vi "Display Results.vi"(8 "error in (no error)":errorcluster, 10 "Results.lvclass":refnum<class "Results.lvclass">, 11 "Operator UI in":refnum<class "Measurement UI.lvclass">) -> (0 "error out":errorcluster, 3 "Operator UI out":refnum<class "Measurement UI.lvclass">)   [LabVIEW 2015, in "Measurement UI.lvlib" / "Measurement UI.lvclass"]
uses:
  Measurement UI.lvclass
  Results/Results.lvclass
  Measurement UI.lvclass/Measurement UI.ctl
  Results/Results.lvclass/Results.ctl
  Accessors/Read Results Listbox.vi
  User Interface/UI.lvclass
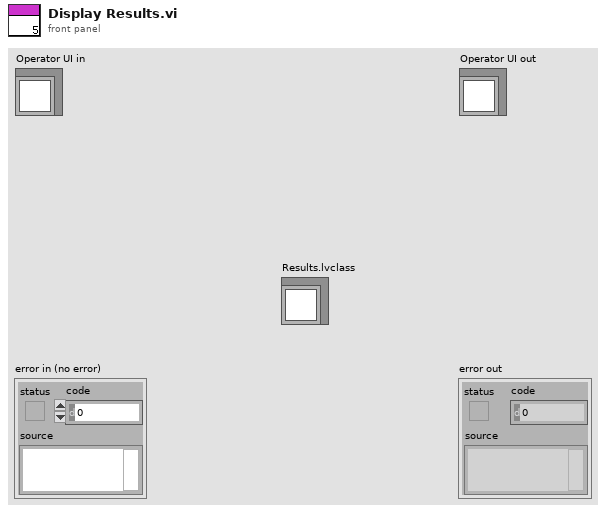
[diagram p1: front panel]
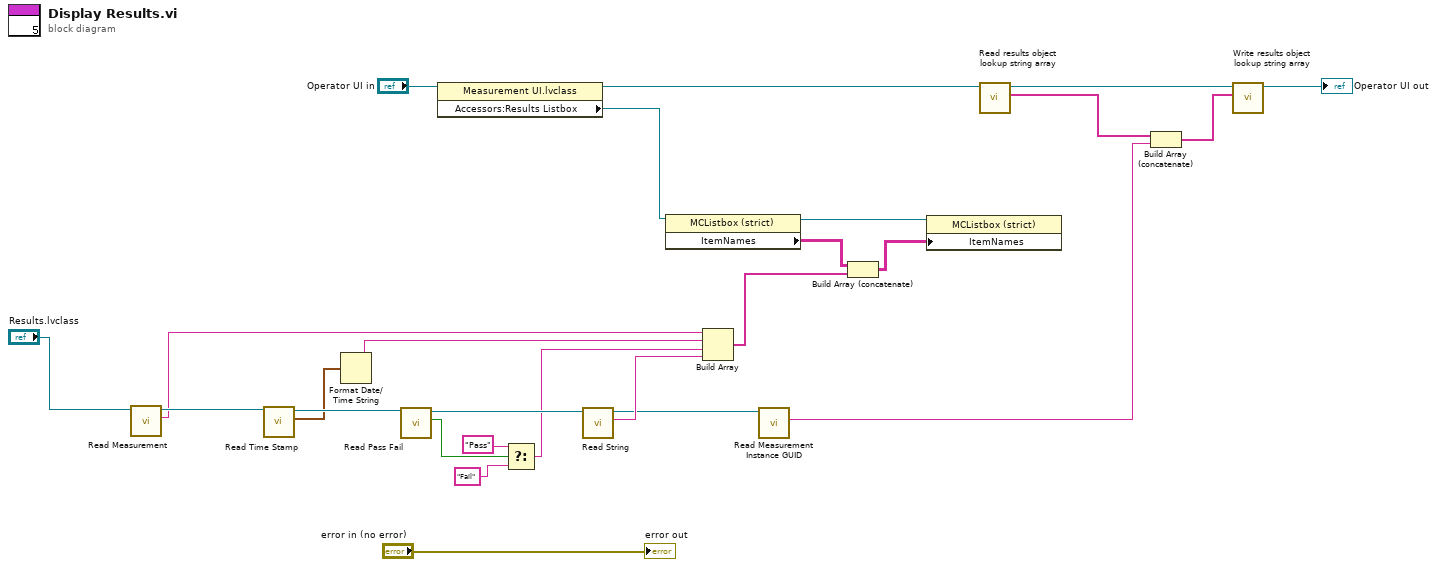
[diagram p0: block diagram]
diagram:
  n1 = call "Read Measurement.vi"("Results in"="Results.lvclass") -> ("Measurement"=w12:string, "Results out"=w13:refnum<class "Results.lvclass">)  [unwired: 8 in, 1 out]
  n2 = call "Read Time Stamp.vi"("Results in"=w13) -> ("Time Stamp"=w9:timestamp, "Results out"=w14:refnum<class "Results.lvclass">)  [unwired: 8 in, 1 out]
  n3 = Format Date/Time String(seconds (now)=w9) -> (date/time string=w10:string)  [unwired: 2 in]
  n4 = call "Read Pass Fail.vi"("Results in"=w14) -> ("Pass Fail"=w18:bool, "Results out"=w19:refnum<class "Results.lvclass">)  [unwired: 8 in, 1 out]
  n5 = property class="Measurement UI.lvclass"(reference="Operator UI in") -> (reference out=w2:refnum<class "Measurement UI.lvclass">, "Accessors:Results Listbox"=w1:refnum<vi>)  [unwired: 1 in, 1 out]
  n6 = Select(t="Pass" ("element"), s=w18, f="Fail" ("element")) -> (s? t:f=w15:string)
  n7 = call "Read String.vi"("Results in"=w19) -> ("String"=w20:string, "Results out"=w4:refnum<class "Results.lvclass">)  [unwired: 8 in, 1 out]
  n8 = property class="MCListbox (strict)"(reference=w1) -> (reference out=w24:refnum<vi>, "ItemNames"=w23:string[][])  [unwired: 1 in, 1 out]
  n9 = Build Array(w12, w10, w15, w20) -> (w21:string[])
  n10 = call "Read Measurement Instance GUID.vi"("Results in"=w4) -> ("Measurement Instance GUID"=w3:string)  [unwired: 8 in, 2 out]
  n11 = Build Array (concatenate)(w23, w21) -> (w22:string[][])
  n12 = property class="MCListbox (strict)"(reference=w24, "ItemNames"=w22) -> ()  [unwired: 1 in, 2 out]
  n13 = call "Read results object lookup string array.vi"("UI in"=w2) -> ("results object lookup string array"=w6:string[], "UI out"=w8:refnum<class "Measurement UI.lvclass">)  [unwired: 8 in, 1 out]
  n14 = Build Array (concatenate)(w6, w3) -> (w5:string[])
  n15 = call "Write results object lookup string array.vi"("results object lookup string array"=w5, "UI in"=w8) -> ("UI out"=→"Operator UI out":refnum<class "Measurement UI.lvclass">)  [unwired: 8 in, 1 out]
  "error out" <- "error in (no error)"
